vi "UART PID to angle against wall.vi"() -> ()   [LabVIEW 2017]
uses:
  <vilib>/myRIO/Instrument Drivers/Onboard IO/UART/typedef/VISA Configuration.ctl
  <vilib>/myRIO/Instrument Drivers/Onboard IO/DIO/typedefs/DIO Reference.ctl
  <vilib>/myRIO/Common/Instrument Driver Framework/Utilities/typedefs/myRIO Generic Hardware Reference.ctl
  <vilib>/myRIO/Common/Instrument Driver Framework/Utilities/typedefs/Hardware Version Enum.ctl
  <vilib>/myRIO/Common/Instrument Driver Framework/Utilities/typedefs/myRIO v1.0 Reference.ctl
  <vilib>/myRIO/Common/Instrument Driver Framework/Utilities/typedefs/Generic FPGA Reference.ctl
  <vilib>/myRIO/Common/Instrument Driver Framework/myRIO v1.0/DIO/typedefs/DIO Channels List.ctl
  <vilib>/myRIO/Common/Instrument Driver Framework/myRIO v1.0/DIO/typedefs/DIO Channels Enum.ctl
  <vilib>/userdefined/High Color/nirio_resource_hc.ctl
  <vilib>/myRIO/Common/Instrument Driver Framework/Utilities/vis/Is FPGA Ref Available.vi
  <vilib>/myRIO/Common/Instrument Driver Framework/myRIO v1.0/DIO/vis/myRIO v1.1 Open DIO.vi
  <vilib>/myRIO/Instrument Drivers/Onboard IO/DIO/vis/Write.vi
  <vilib>/myRIO/Common/Instrument Driver Framework/Utilities/vis/Validate Channels.vi
  <vilib>/myRIO/Common/Instrument Driver Framework/myRIO v1.0/DIO/vis/myRIO v1.0 Reserve DIO.vi
  <vilib>/myRIO/Common/Instrument Driver Framework/myRIO v1.0/Resource Manager/vis/myRIO v1.0 Reserve Channel List.vi
  <vilib>/myRIO/Common/Instrument Driver Framework/myRIO v1.0/DIO/vis/myRIO v1.0 Build MUX Configuration DIO.vi
  <vilib>/myRIO/Common/Instrument Driver Framework/myRIO v1.0/Resource Manager/vis/myRIO v1.0 Reserve Channel.vi
  <vilib>/myRIO/Common/Instrument Driver Framework/myRIO v1.0/Resource Manager/vis/myRIO v1.0 Unreserve Channel.vi
  <vilib>/myRIO/Common/Instrument Driver Framework/myRIO v1.0/Resource Manager/vis/myRIO v1.0 Create Configuration List.vi
  <vilib>/myRIO/Common/Instrument Driver Framework/myRIO v1.0/Resource Manager/vis/myRIO v1.0 Build Mutex Name.vi
  <vilib>/Utility/VariantDataType/GetNumericInfo.vi
  <vilib>/Utility/error.llb/Error Cluster From Error Code.vi
  <vilib>/myRIO/Common/Instrument Driver Framework/myRIO v1.0/myRIO v1.1 Open.vi
  <vilib>/myRIO/Common/Instrument Driver Framework/Utilities/vis/IO Manager.vi
  <vilib>/myRIO/Common/Instrument Driver Framework/Utilities/vis/Configuration Manager.vi
  <vilib>/myRIO/Common/Instrument Driver Framework/myRIO v1.0/Resource Manager/vis/myRIO v1.0 Configure IO.vi
  <vilib>/myRIO/Common/Instrument Driver Framework/myRIO v1.0/myRIO v1.0 Close.vi
  <vilib>/myRIO/Common/Instrument Driver Framework/myRIO v1.0/DIO/vis/myRIO v1.0 Write DIO.vi
  <vilib>/Instr/_visa.llb/VISA Configure Serial Port (Instr).vi
  <vilib>/myRIO/Express VI/Onboard Devices/LED/LED Express VI.xnode
  <vilib>/myRIO/Instrument Drivers/Onboard IO/DIO/vis/myRIO DIO Open.xnode
  <vilib>/myRIO/Instrument Drivers/Onboard IO/DIO/DIO.lvlib
  <vilib>/myRIO/Instrument Drivers/Onboard IO/UART/UART.lvlib
panel:
  in  "VISA resource name in":refnum<visa-resource-name>="ASRL3::INSTR"
  out "dt":u32
  in  "stop":bool
  out "com i":i32
  out "result":bool
  out "Loop num":i32
  out "timeout (10sec)":u32
  in  "Initial delay (ms)":u32=1000
  in  "number of variables":i32=3
  out "Array":string[](array[string])
  in  "input cluster":T1={"baud rate (9600)"=115200, "data bits (8)"=8, "parity (0:none)"=enum."None", "stop bits (10: 1 bit)"=10, "flow control (0:none)"=0, "termination char\n(0xA = '\\n' = LF) "=10, "Enable Termination\nChar (T)"=TRUE, "timeout (10sec)"=1000} {"termination char\n(0xA = '\\n' = LF)" format="%.0x"; "flow control (0:none)" items=["None", "XON/XOFF", "RTS/CTS", "XON/XOFF & RTS/CTS", "DTR/DSR", "XON/XOFF & DTR/DSR"]; "stop bits (10: 1 bit)" items=["1.0"=10, "1.5"=15, "2.0"=20]; "data bits (8)" min=5 max=8 step=1}
  out "error out":errorcluster
  out "Characters Read":string
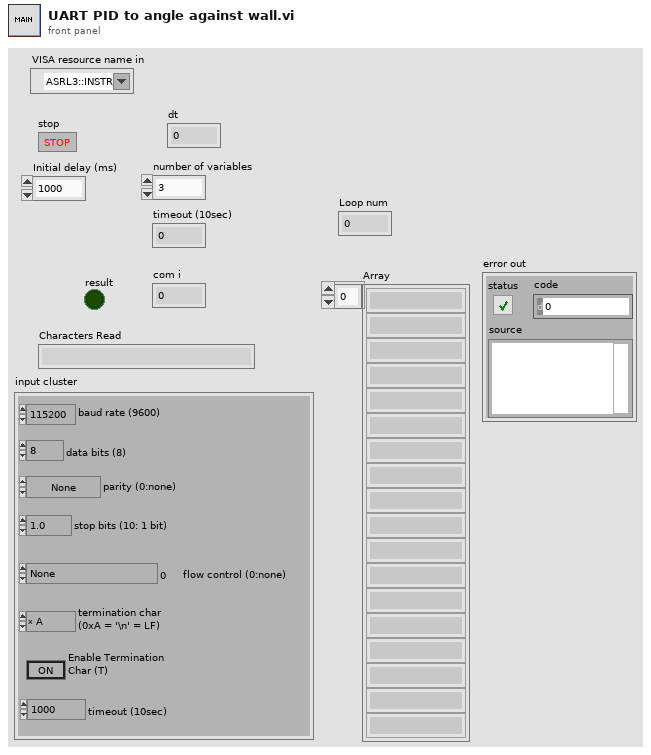
[diagram p1: front panel]
types:
  T1 = typedef "UART.lvlib/VISA Configuration.ctl" = cluster{"baud rate (9600)":u32, "data bits (8)":u16, "parity (0:none)":enum16{"None", "Odd", "Even", "Mark", "Space"}, "stop bits (10: 1 bit)":u16, "flow control (0:none)":u16, "termination char\n(0xA = '\\n' = LF) ":u8, "Enable Termination\nChar (T)":bool, "timeout (10sec)":u32}
  T2 = typedef "DIO.lvlib/DIO Reference.ctl" = cluster{"myRIO Reference":T3, "DIO Channels List":T7}
  T3 = typedef "myRIO Generic Hardware Reference.ctl" = cluster{"myRIO Model":T4, "myRIO Hardware Reference":T5}
  T4 = typedef "Hardware Version Enum.ctl" = enum16{"Unknown", "myRIO-1900", "myRIO-1950", "roboRIO", "NI ELVIS RIO CM"}
  T5 = typedef "myRIO v1.0 Reference.ctl" = cluster{"Generic FPGA Reference":T6, "Allow multiple opens":bool}
  T6 = typedef "Generic FPGA Reference.ctl" = refnum<k20>
  T7 = typedef "DIO Channels List.ctl" = T8[]
  T8 = typedef "DIO Channels Enum.ctl" = enum16{"Not Connected", "C/DIO0", "C/DIO1", "C/DIO2", "C/DIO3", "C/DIO4", "C/DIO5", "C/DIO6", "C/DIO7", "A/DIO0", "A/DIO1", "A/DIO2", "A/DIO3", "A/DIO4", "A/DIO5", "A/DIO6", "A/DIO7", "A/DIO8", "A/DIO9", "A/DIO10", "A/DIO11", "A/DIO12", "A/DIO13", "A/DIO14", "A/DIO15", "B/DIO0", "B/DIO1", "B/DIO2", "B/DIO3", "B/DIO4", "B/DIO5", "B/DIO6", "B/DIO7", "B/DIO8", "B/DIO9", "B/DIO10", "B/DIO11", "B/DIO12", "B/DIO13", "B/DIO14", "B/DIO15", "LED0", "LED1", "LED2", "LED3", "Button0", "DIO/DIO0", "DIO/DIO1", "DIO/DIO2", "DIO/DIO3", "DIO/DIO4", "DIO/DIO5", "DIO/DIO6", "DIO/DIO7", "DIO/DIO8", "DIO/DIO9", "SPI/CS0", "SPI/CS1", "SPI/CS2", "SPI/CS3", "LED RADIO (Green)", "LED RADIO (Red)", "LED COMM (Green)", "LED COMM (Red)", "LED MODE (Green)", "LED MODE (Red)"}
  T9 = typedef "nirio_resource_hc.ctl" = tag
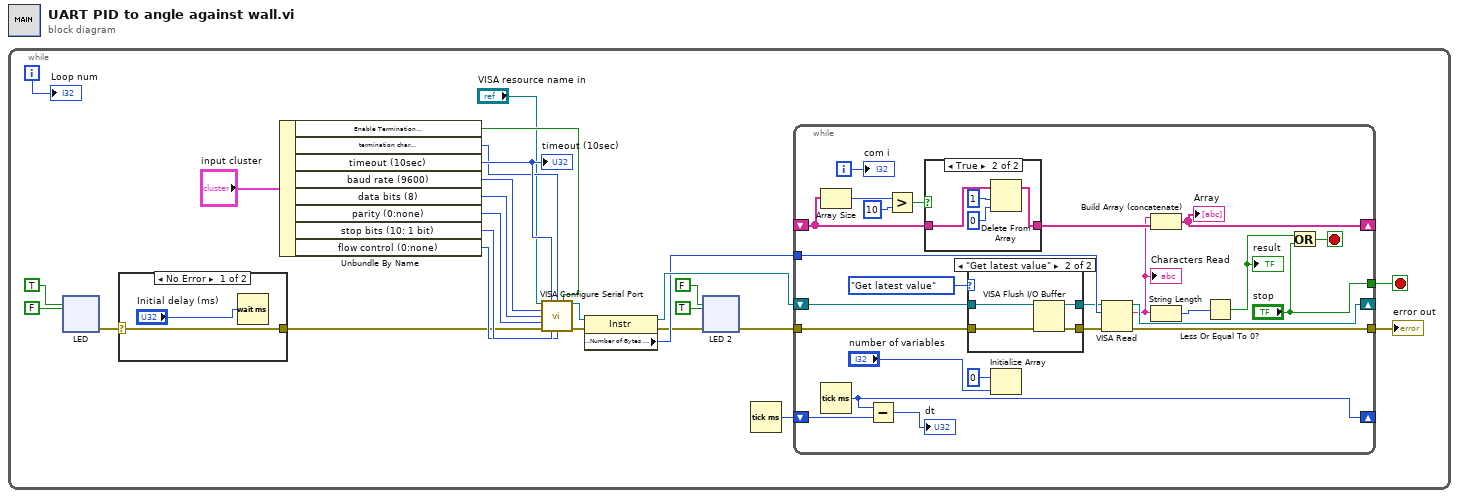
[diagram p0: block diagram]
diagram:
  n1 = while {
    i -> [w6]
    stop <- w2 stop-if-true
    n2 = xnode "LED"("LED0"=TRUE, "LED3"=FALSE ("LED1")) -> ("error out"=w12:errorcluster)  [unwired: 1 in]
    n3 = case shown="No Error" w12 {
      selector: w12 -> [w99 w101]
      tunnel: [w99 w101] -> w3
      frame No Error {
        n4 = Wait (ms)(milliseconds to wait="Initial delay (ms)") -> ()  [unwired: 1 out]
      }
      frame Error {
      }
    }
    n5 = Unbundle By Name("input cluster") -> ("Enable Termination\nChar (T)"=w19:bool, "termination char\n(0xA = '\\n' = LF)"=w20:u8, "timeout (10sec)"=w21:u32, "baud rate (9600)"=w26:u32, "data bits (8)"=w25:u16, "parity (0:none)"=w24:enum16{"None", "Odd", "Even", "Mark", "Space"}, "stop bits (10: 1 bit)"=w23:u16, "flow control (0:none)"=w22:u16)
    "timeout (10sec)" <- w21
    n6 = call-poly "VISA Configure Serial Port"("VISA resource name"="VISA resource name in", "timeout (10sec)"=w21, "termination char\n(0xA = '\\n' = LF)"=w20, "Enable Termination\nChar (T)"=w19, "baud rate (9600)"=w26, "data bits (8)"=w25, "parity (0:none)"=w24, "error in (no error)"=w3, "stop bits (10: 1 bit)"=w23, "flow control (0:none)"=w22) -> ("VISA resource name out"=w15:refnum<visa-resource-name>, "error out"=w16:errorcluster)  [unwired: 4 in]
    n7 = property class="Instr"(reference=w15, error in=w16) -> (reference out=w14:refnum<visa-resource-name>, error out=w10:errorcluster, "Serial Settings:Number of Bytes at Serial Port"=w13:u32)
    n8 = xnode "LED 2"("error in (no error)"=w10, "LED0"=FALSE, "LED3"=TRUE) -> ("error out"=w5:errorcluster)
    n9 = Tick Count (ms)() -> (millisecond timer value=w4:u32)
    n10 = while {
      tunnel: w13 -> [w126]
      shift-right: [w122] -> _
      shift-left: w14 -> [w125]
      shift-right: [w103] -> _
      shift-left: w4 -> [w104]
      shift-right: [w120] -> _
      shift-left: _ -> [w116]
      tunnel: w5 -> [w110]
      tunnel: ["stop"] -> w2
      tunnel: [w105] -> w1
      i -> [w111]
      stop <- w106 stop-if-true
      n11 = Array Size(array=w116) -> (size(s)=w119:i32)
      n12 = Tick Count (ms)() -> (millisecond timer value=w103:u32)
      n13 = Subtract(x=w103, y=w104) -> (x-y=→"dt":u32)
      n14 = Greater?(x=w119, y=10) -> (0:w117:bool)
      n15 = case shown="True" w117 {
        tunnel: w116 -> [w127 w131]
        tunnel: [w127 w128] -> w115
        frame False {
        }
        frame True {
          n16 = Delete From Array(array=w131, length=1, index=0) -> (array with subset deleted=w128:string[])  [unwired: 1 out]
        }
      }
      n17 = case shown="\"Get latest value\"" enum16{"Read all", "Get latest value"}."Get latest value" {
        tunnel: w125 -> [w133 w137]
        tunnel: w110 -> [w132 w136]
        tunnel: [w132 w134] -> w124
        tunnel: [w133 w135] -> w123
        frame "Read all", Default {
        }
        frame "Get latest value" {
          n18 = VISA Flush I/O Buffer(VISA resource name=w137, error in (no error)=w136) -> (VISA resource name out=w135:refnum<visa-resource-name>, error out=w134:errorcluster)  [unwired: 1 in]
        }
      }
      n19 = Initialize Array(0 ("element"), "number of variables") -> ()  [unwired: 1 out]
      n20 = VISA Read(VISA resource name=w123, byte count=w126, error in (no error)=w124) -> (VISA resource name out=w122:refnum<visa-resource-name>, read buffer=w112:string, error out=w105:errorcluster)  [unwired: 1 out]
      "Characters Read" <- w112
      n21 = Build Array (concatenate)(w112, w115) -> (w120:string[])
      "Array" <- w120
      n22 = String Length(string=w112) -> (length=w109:i32)
      n23 = Less Or Equal To 0?(x=w109) -> (x <= 0?=w107:bool)
      "result" <- w107
      n24 = Or(x=w107, y="stop") -> (x .or. y?=w106:bool)
      "com i" <- w111
    }
    "error out" <- w1
    "Loop num" <- w6
  }
